vi "ColorCodeRotation.vi"(0 "Output":dbl) -> ()   [LabVIEW 2019]
uses:
  <vilib>/Rock Robotics/WPI/ThirdParty/Phoenix-LabVIEW/Motor Controller/Controls/CTRE_Phoenix_MotorControl_ControlMode.ctl
panel:
  in  "?":bool
  out "Color Counter":i32
  in  "Blue Calibration":cluster{"R":dbl, "G":dbl, "B":dbl}={"R"=0.143, "G"=0.427, "B"=0.429}
  in  "Green Calibration":cluster{"R":dbl, "G":dbl, "B":dbl}={"R"=0.197, "G"=0.561, "B"=0.24}
  in  "Red Calibration":cluster{"R":dbl, "G":dbl, "B":dbl}={"R"=0.561, "G"=0.323, "B"=0.114}
  in  "Yellow Calibration":cluster{"R":dbl, "G":dbl, "B":dbl}={"R"=0.361, "G"=0.524, "B"=0.113}
  out "Color":u32(colorbox)
  out "Matched Color Name":string
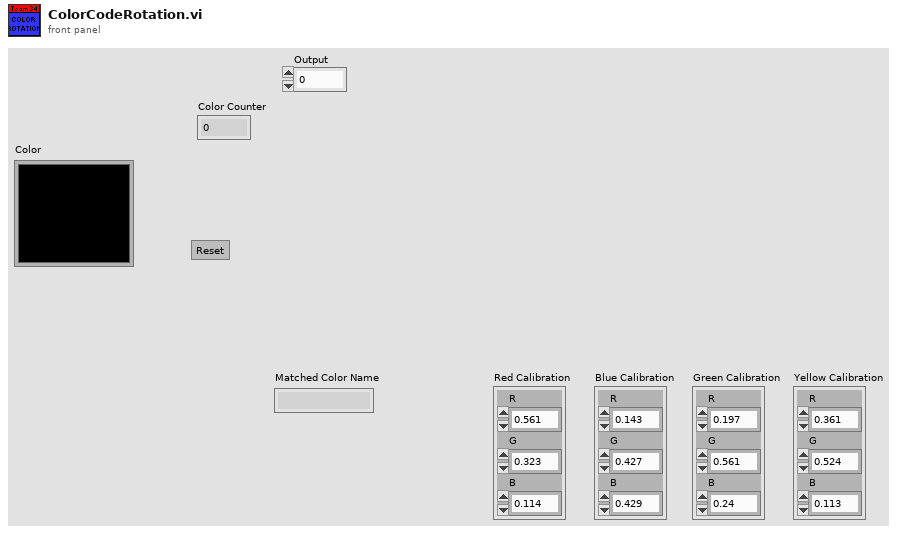
[diagram p1: front panel]
types:
  T1 = typedef "Color Sensor V3 DevRef.ctl" = cluster{"I2CDevRef":T2}
  T2 = typedef "WPI_I2CDevRef.ctl" = cluster{"DevStatus":errorcluster, "Device Address":u8, "Handle":i32, "I2C Bus":T3}
  T3 = typedef "i2c_bus.ctl" = enum16{"I2C On-Board", "I2C MXP", "Invalid"}
  T4 = typedef "CTRE_Phoenix_MotorControl_ControlMode.ctl" = u16
  T5 = typedef "WPI_MotorControlDeviceRef.ctl" = cluster{"DeviceStatus":errorcluster, "Type":T6, "PWM":cluster{"PWM Channel":T7, "DeadBand":T8}, "CAN":cluster{"Device Number":u8, "SetOutput VI Ref":variant, "GetOutput VI Ref":variant, "Enable VI Ref":variant, "Disable VI Ref":variant, "Data":variant}, "Invert":bool, "DIO PWM":cluster{"PWM \"Enable\" Channel":T7, "DIOChannel":T9, "PWM Rate":dbl}}
  T6 = typedef "WPI_MotorControlType.ctl" = enum16{"PWM", "CAN", "DIO PWM"}
  T7 = typedef "FPGA_DIOPWMChannel.ctl" = enum8{"PWM 0", "PWM 1", "PWM 2", "PWM 3", "PWM 4", "PWM 5", "PWM 6", "PWM 7", "PWM 8", "PWM 9", "PWM MXP 0", "PWM MXP 1", "PWM MXP 2", "PWM MXP 3", "PWM MXP 4", "PWM MXP 5", "PWM MXP 6", "PWM MXP 7", "PWM MXP 8", "PWM MXP 9", "Invalid"}
  T8 = typedef "WPI_PWMDeadband.ctl" = cluster{"Name":string, "maxPositivePwm":i32, "minPositivePwm":i32, "centerPwm":i32, "maxNegativePwm":i32, "minNegativePwm":i32, "angularRange":u16}
  T9 = typedef "FPGA_DIOChannel.ctl" = enum8{"DIO 0", "DIO 1", "DIO 2", "DIO 3", "DIO 4", "DIO 5", "DIO 6", "DIO 7", "DIO 8", "DIO 9", "DIO MXP 0", "DIO MXP 1", "DIO MXP 2", "DIO MXP 3", "DIO MXP 4", "DIO MXP 5", "DIO MXP 6", "DIO MXP 7", "DIO MXP 8", "DIO MXP 9", "DIO MXP 10", "DIO MXP 11", "DIO MXP 12", "DIO MXP 13", "DIO MXP 14", "DIO MXP 15", "SPI Port CS1", "SPI Port CS2", "SPI Port CS3", "SPI Port MISO", "SPI Port MOSI", "Invalid"}
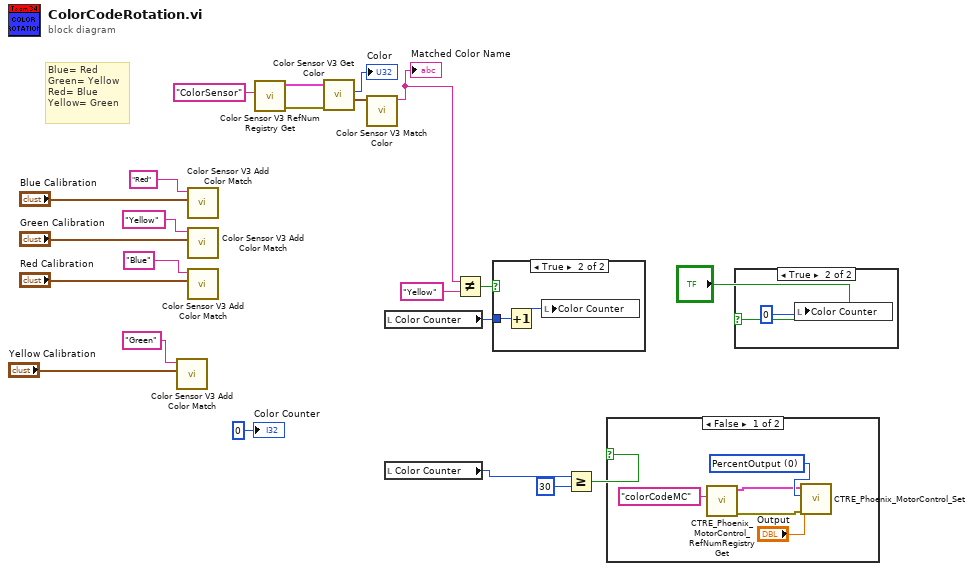
[diagram p0: block diagram]
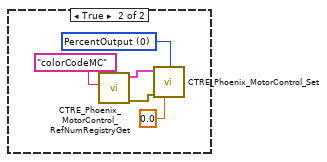
[diagram p2: hidden frame]
diagram:
  # "Blue= Red\nGreen= Yellow\nRed= Blue \nYellow= Green"
  n1 = call <vilib>:"Color Sensor V3 Add Color Match.vi"("Color"="Yellow Calibration", "Name"="Green") -> ()  [unwired: 10 in]
  n2 = call <vilib>:"Color Sensor V3 Add Color Match.vi"("Color"="Blue Calibration", "Name"="Red") -> ()  [unwired: 10 in]
  n3 = call <vilib>:"Color Sensor V3 Add Color Match.vi"("Color"="Green Calibration", "Name"="Yellow") -> ()  [unwired: 10 in]
  n4 = call <vilib>:"Color Sensor V3 Add Color Match.vi"("Color"="Red Calibration", "Name"="Blue") -> ()  [unwired: 10 in]
  n5 = call <vilib>:"Color Sensor V3 RefNum Registry Get.vi"("refnum name"="ColorSensor") -> ("error out"=w3:errorcluster, "ColorSensorDevRef"=w4:T1)  [unwired: 9 in]
  n6 = call <vilib>:"Color Sensor V3 Get Color.vi"("error in (no error)"=w3, "ColorSensorDevRef"=w4) -> ("Normalized Color"=w14:cluster{"R":dbl, "G":dbl, "B":dbl}, "Color"=→"Color":u32)  [unwired: 6 in, 2 out]
  n7 = call <vilib>:"Color Sensor V3 Match Color.vi"("Measured Color"=w14) -> ("Matched Color Name"=w12:string)  [unwired: 8 in, 2 out]
  "Matched Color Name" <- w12
  n8 = local read "Color Counter"() -> (w10:i32)
  n9 = local read "Color Counter"() -> (w6:i32)
  n10 = Not Equal?(x=w12, y="Yellow") -> (x != y?=w11:bool)
  n11 = case shown="True" w11 {
    tunnel: w10 -> [_ w24]
    frame False {
    }
    frame True {
      n12 = Increment(x=w24) -> (x+1=w23:i32)
      n13 = local write "Color Counter"(w23) -> ()
    }
  }
  n14 = Greater Or Equal?(x=w6, y=30) -> (x >= y?=w7:bool)
  n15 = case shown="False" w7 {
    frame False {
      w29 = T4 0 items=["PercentOutput"=0, "Position"=1, "Velocity"=2, "Current"=3, "Follower"=5, "MotionProfile"=6, "MotionMagic"=7, "MotionProfileArc"=10, "Disabled"=15] ("Control Mode")
      n16 = call <vilib>:"CTRE_Phoenix_MotorControl_RefNumRegistryGet.vi"("refnum name"="colorCodeMC") -> ("error out"=w27:errorcluster, "PhoenixMotorControlDevRef"=w28:T5)  [unwired: 9 in]
      n17 = call <vilib>:"CTRE_Phoenix_MotorControl_Set.vi"("error in (no error)"=w27, "Output"="Output", "Control Mode"=w29, "PhoenixMotorControlDevRef"=w28) -> ()  [unwired: 6 in, 2 out]
    }
    frame True {
      w34 = T4 0 items=["PercentOutput"=0, "Position"=1, "Velocity"=2, "Current"=3, "Follower"=5, "MotionProfile"=6, "MotionMagic"=7, "MotionProfileArc"=10, "Disabled"=15] ("Control Mode")
      n18 = call <vilib>:"CTRE_Phoenix_MotorControl_RefNumRegistryGet.vi"("refnum name"="colorCodeMC") -> ("error out"=w31:errorcluster, "PhoenixMotorControlDevRef"=w32:T5)  [unwired: 9 in]
      n19 = call <vilib>:"CTRE_Phoenix_MotorControl_Set.vi"("error in (no error)"=w31, "Output"=0.0, "Control Mode"=w34, "PhoenixMotorControlDevRef"=w32) -> ()  [unwired: 6 in, 2 out]
    }
  }
  n20 = case shown="True" "?" {
    frame False {
    }
    frame True {
      n21 = local write "Color Counter"(0 ("Numeric")) -> ()
    }
  }
  "Color Counter" <- 0 ("Color Counter")
